vi "measVoltGlobVars.vi"() -> ()   [LabVIEW 2014]
uses:
  Controls/measVoltState.ctl
panel:
  in  "measVoltState":T1
  out "timedOutWhileHandshake":bool
  in  "measVoltTimeout(10ns)":i32 caption="measVoltTimeout(25ns)"
  in  "measVoltPulseLength(25ns)":i32
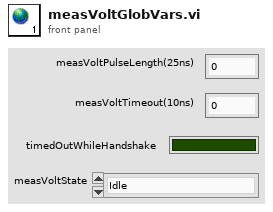
[diagram p1: front panel]
types:
  T1 = typedef "measVoltState.ctl" = enum16{"Idle", "sendMeasRequest", "waitUntilDone", "done"}
diagram:
